vi "global_notaus.vi"() -> ()   [LabVIEW 2013]
panel:
  in  "Notaus":bool
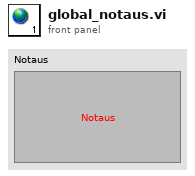
[diagram p1: front panel]
diagram:
